vi "Read Marker.vi"(8 "error in (no error)":errorcluster, 11 "SpecAnBase in":refnum<class "SpecAnBase.lvclass">) -> (0 "error out":errorcluster, 2 "Marker":T1={"MarkerEnabled"=FALSE, "MarkerThreshold"=0.0, "PeakExcursion"=0.0, "SignalTrackEnabled"=FALSE, "MarkerPosition"=0.0, "Instrument Setting (Frequency Center)"=1, "Marker search (Minimum)"=2, "ActiveMarker"="", "MarkerFrequencyCounter"=FALSE, "FrequencyCounterResolution"=0.0} {"Marker search (Minimum)" items=["Highest"=1, "Next Peak"=3, "Next Peak Left"=4, "Next Peak Right"=5, "Minimum"=2]; "Instrument Setting (Frequency Center)" items=["Frequency Start"=3, "Frequency Stop"=4, "Frequency Center"=1, "Frequency Span"=2, "Reference Level"=5]}, 3 "SpecAnBase out":refnum<class "SpecAnBase.lvclass">)   [LabVIEW 2018, in "SpecAnPlugins.lvlib" / "SpecAnBase.lvclass"]
uses:
  SpecAnBase.lvclass
  Typedefs/Markers.ctl
  SpecAnBase.lvclass/SpecAnBase.ctl
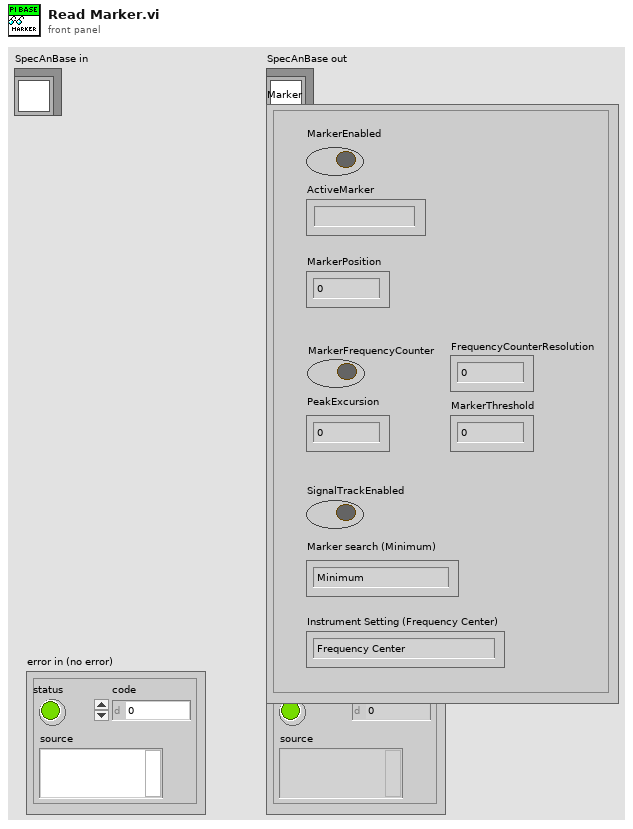
[diagram p1: front panel]
types:
  T1 = typedef "SpecAnPlugins.lvlib/SpecAnBase.lvclass/Markers.ctl" = cluster{"MarkerEnabled":bool, "MarkerThreshold":dbl, "PeakExcursion":dbl, "SignalTrackEnabled":bool, "MarkerPosition":dbl, "Instrument Setting (Frequency Center)":i32, "Marker search (Minimum)":i32, "ActiveMarker":string, "MarkerFrequencyCounter":bool, "FrequencyCounterResolution":dbl}
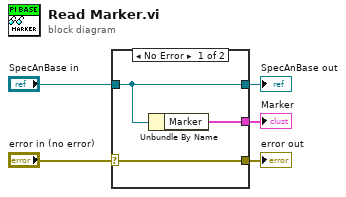
[diagram p0: block diagram]
diagram:
  n1 = case shown="No Error" "error in (no error)" {
    selector: "error in (no error)" -> [w8 w9]
    tunnel: [w8 w9] -> w4
    tunnel: [w7 w10] -> w2
    tunnel: "SpecAnBase in" -> [w7 w10]
    tunnel: [w6 _] -> w1
    frame No Error {
      n2 = Unbundle By Name(w7) -> ("Marker"=w6:T1)
    }
    frame Error {
    }
  }
  "error out" <- w4
  "SpecAnBase out" <- w2
  "Marker" <- w1
